vi "AddPyExtension.vi"(11 "selected path":path) -> (3 "dup file":path)   [LabVIEW 2019]
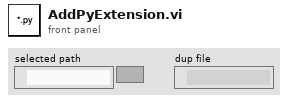
[diagram p1: front panel]
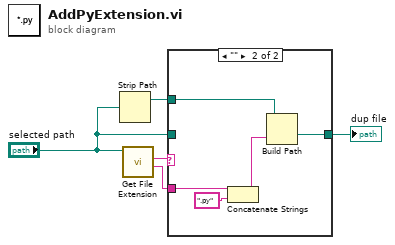
[diagram p0: block diagram]
diagram:
  n1 = Strip Path(path="selected path") -> (stripped path=w3:path)  [unwired: 1 out]
  n2 = call <vilib>:"Get File Extension.vi"("file"="selected path") -> ("filename without extension"=w4:string, "lowercase file extension"=w5:string)  [unwired: 6 in, 3 out]
  n3 = case shown="\"\"" w5 {
    tunnel: w4 -> [_ w11]
    tunnel: w3 -> [_ w9]
    tunnel: [w6 w7] -> w2
    tunnel: "selected path" -> [w6 _]
    frame Default {
    }
    frame "" {
      n4 = Concatenate Strings(w11, ".py" ("string")) -> (w8:string)
      n5 = Build Path(base path=w9, name or relative path=w8) -> (appended path=w7:path)
    }
  }
  "dup file" <- w2
